vi "Choreo_SwerveSample_GetPose.vi"(11 "ChoreoSwerveSample":T4) -> (3 "Pose":T1 {"ROTATION"."SIN" format="%13.4f"; "ROTATION"."COS" format="%13.4f"; "ROTATION"."VALUE" format="%13.4f"; "TRANSLATION"."Y" format="%14.3f"; "TRANSLATION"."X" format="%14.3f"})   [LabVIEW 2019, in "ChoreoLib.lvlib"]
doc: "Returns the pose at this sample.\n\nInputs:\n -- ChoreoSwerveSample - cluster - Swerve sample.\n \nOutputs: \n -- Pose - Pose2d - The pose at this sample."
uses:
  ChoreoLib.lvlib
  TypeDef/ChoreoSwerveSample.ctl
  <vilib>/Rock Robotics/WPI/ThirdParty/JAS_Junk/TrajLib/TypeDef/POSE2D.ctl
  <vilib>/Rock Robotics/WPI/ThirdParty/JAS_Junk/TrajLib/TypeDef/TRANSLATION2D.ctl
  <vilib>/Rock Robotics/WPI/ThirdParty/JAS_Junk/TrajLib/TypeDef/ROTATION2D.ctl
  <vilib>/Rock Robotics/WPI/ThirdParty/JAS_Junk/TrajLib/Rotation2d_CreateAngle.vi
  <vilib>/Rock Robotics/WPI/ThirdParty/JAS_Junk/TrajLib/Translation2d_Create.vi
  <vilib>/Rock Robotics/WPI/ThirdParty/JAS_Junk/TrajLib/Trajectory_Library.lvlib
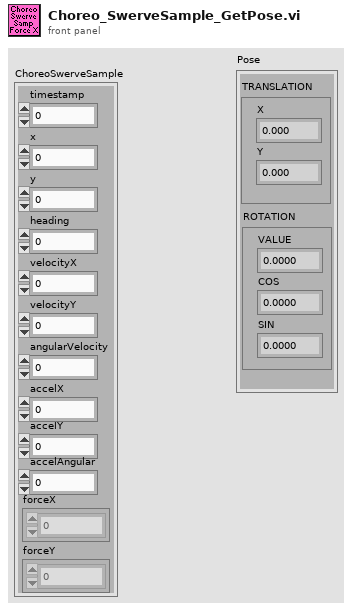
[diagram p1: front panel]
types:
  T1 = typedef "Trajectory_Library.lvlib/POSE2D.ctl" = cluster{"TRANSLATION":T2, "ROTATION":T3}
  T2 = typedef "Trajectory_Library.lvlib/TRANSLATION2D.ctl" = cluster{"X":dbl, "Y":dbl}
  T3 = typedef "Trajectory_Library.lvlib/ROTATION2D.ctl" = cluster{"VALUE":dbl, "COS":dbl, "SIN":dbl}
  T4 = typedef "ChoreoLib.lvlib/ChoreoSwerveSample.ctl" = cluster{"timestamp":dbl, "x":dbl, "y":dbl, "heading":dbl, "velocityX":dbl, "velocityY":dbl, "angularVelocity":dbl, "accelX":dbl, "accelY":dbl, "accelAngular":dbl, "forceX":dbl[], "forceY":dbl[]}
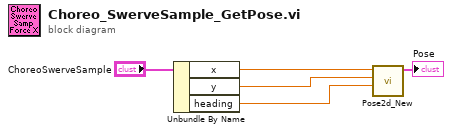
[diagram p0: block diagram]
diagram:
  n1 = Unbundle By Name("ChoreoSwerveSample") -> ("x"=w4:dbl, "y"=w3:dbl, "heading"=w2:dbl)
  n2 = call <vilib>:"Pose2d_New.vi"("Heading"=w2, "Y"=w3, "X"=w4) -> ("out POSe"=→"Pose":T1)  [unwired: 8 in]
